vi "Dialog Box - Three Button.vi"(5 "Key Focus":enum16{"None", "1", "2", "3"}(ring), 6 "Button Text":T1={"Button 1"="Yes", "Button 2"="No", "Button 3"="Cancel"}, 7 "Timeout (Seconds)":i16=-1, 8 "error in (no error)":errorcluster, 11 "Text":string) -> (0 "error out":errorcluster, 1 "Button 3":bool, 2 "Button 2":bool, 3 "Button 1":bool, 4 "Timeout":bool)   [LabVIEW 2011]
doc: "Displays a simple two button dialog box.\n\nA timeout can be set. If no timeout is defined then the dialog will wait forever.\nThe text for each button can be set.\nEither button can receive key focus."
panel:
  in  "Button Three":bool
  in  "Button Two":bool
  in  "Button One":bool
  out "String":string
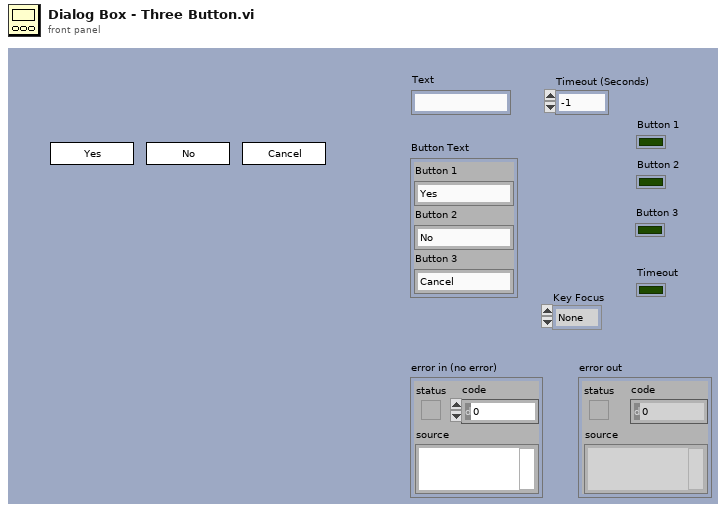
[diagram p1: front panel]
types:
  T1 = cluster{"Button 1":string, "Button 2":string, "Button 3":string}
  T2 = enum32{"Invalid", "Default", "Floating", "Floating/Auto-Hide", "Modal"}
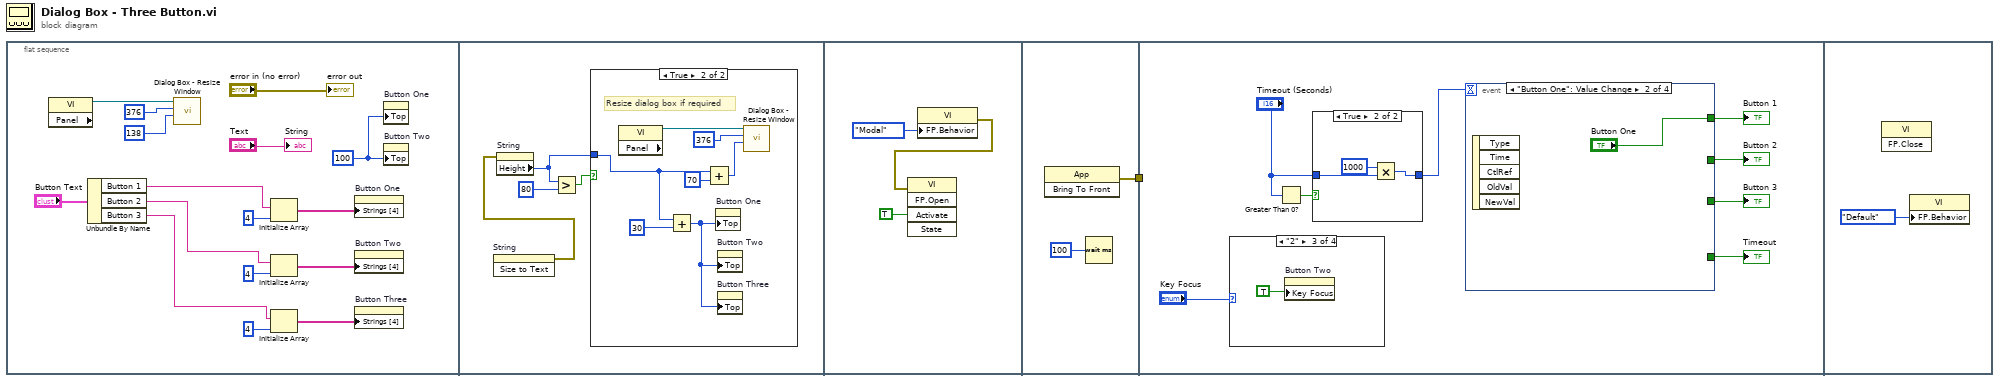
[diagram p0: block diagram]
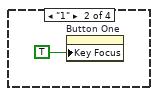
[diagram p4: hidden frame]
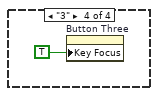
[diagram p5: hidden frame]
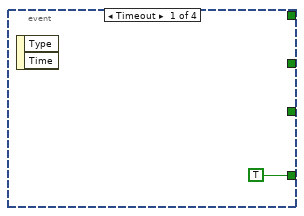
[diagram p6: hidden frame]
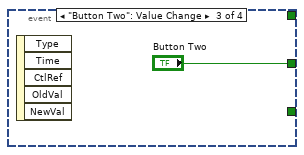
[diagram p7: hidden frame]
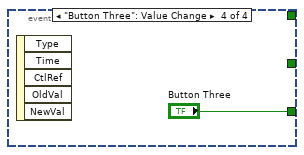
[diagram p8: hidden frame]
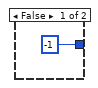
[diagram p9: hidden frame]
diagram:
  n1 = flat-sequence {
    tunnel: [w33] -> w1
    tunnel: w1 -> [_]
    frame #0 {
      w8 = 100 ("Position:Top")
      n2 = property class="VI" props=["Panel"]() -> (reference out=w11:refnum<vi>)  [unwired: 2 in, 2 out]
      n3 = Unbundle By Name("Button Text") -> ("Button 1"=w5:string, "Button 2"=w4:string, "Button 3"=w3:string)
      n4 = call "Dialog Box - Resize Window.vi"("Height"=i16 138, "Width"=i16 376, "reference"=w11) -> ()  [unwired: 8 in, 1 out]
      n5 = Initialize Array(w5, 4 ("dimension size")) -> (w12:string[])
      n6 = Initialize Array(w4, 4 ("dimension size")) -> (w13:string[])
      n7 = Initialize Array(w3, 4 ("dimension size")) -> (w2:string[])
      n8 = property on="Button One" class="Bool"("Strings [4]"=w12) -> ()  [unwired: 2 in, 2 out]
      n9 = property on="Button Two" class="Bool"("Strings [4]"=w13) -> ()  [unwired: 2 in, 2 out]
      n10 = property on="Button Three" class="Bool"("Strings [4]"=w2) -> ()  [unwired: 2 in, 2 out]
      n11 = property on="Button One" class="Bool"("Top"=w8) -> ()  [unwired: 2 in, 2 out]
      n12 = property on="Button Two" class="Bool"("Top"=w8) -> ()  [unwired: 2 in, 2 out]
      "String" <- "Text"
      "error out" <- "error in (no error)"
    }
    frame #1 {
      n13 = invoke on="String" class="Str" method="Size to Text"() -> (error out=w21:errorcluster)  [unwired: 3 in, 2 out]
      n14 = property on="String" class="Str"(error in=w21) -> ("Height"=w20:u32)  [unwired: 1 in, 2 out]
      n15 = Greater?(x=w20, y=u32 80) -> (0:w19:bool)
      n16 = case shown="True" w19 {
        tunnel: w20 -> [_ w24]
        frame False {
        }
        frame True {
          # "Resize dialog box if required"
          n17 = property class="VI" props=["Panel"]() -> (reference out=w28:refnum<vi>)  [unwired: 2 in, 2 out]
          n18 = Add(x=w24, y=u32 30) -> (x+y=w22:u32)
          n19 = Add(x=w24, y=u32 70) -> (x+y=w26:u32)
          n20 = property on="Button One" class="Bool"("Top"=w22) -> ()  [unwired: 2 in, 2 out]
          n21 = property on="Button Two" class="Bool"("Top"=w22) -> ()  [unwired: 2 in, 2 out]
          n22 = property on="Button Three" class="Bool"("Top"=w22) -> ()  [unwired: 2 in, 2 out]
          n23 = call "Dialog Box - Resize Window.vi"("Height"=w26, "Width"=i16 376, "reference"=w28) -> ()  [unwired: 8 in, 1 out]
        }
      }
    }
    frame #2 {
      n24 = property class="VI"("FP.Behavior"=T2."Modal" ("Front Panel Window:Behavior")) -> (error out=w29:errorcluster)  [unwired: 2 in, 1 out]
      n25 = invoke class="VI" method="FP.Open"(error in=w29, "Activate"=TRUE ("Activate?")) -> ()  [unwired: 3 in, 5 out]
    }
    frame #3 {
      n26 = invoke class="App" method="Bring To Front"() -> (error out=w33:errorcluster)  [unwired: 3 in, 2 out]
      n27 = Wait (ms)(milliseconds to wait=u32 100) -> ()  [unwired: 1 out]
    }
    frame #4 {
      n28 = case shown="\"2\"" "Key Focus" {
        frame "None" {
        }
        frame "1" {
          n29 = property on="Button One" class="Bool"("Key Focus"=TRUE) -> ()  [unwired: 2 in, 2 out]
        }
        frame "2" {
          n30 = property on="Button Two" class="Bool"("Key Focus"=TRUE) -> ()  [unwired: 2 in, 2 out]
        }
        frame "3" {
          n31 = property on="Button Three" class="Bool"("Key Focus"=TRUE) -> ()  [unwired: 2 in, 2 out]
        }
      }
      n32 = Greater Than 0?(x="Timeout (Seconds)") -> (x > 0?=w40:bool)
      n33 = case shown="True" w40 {
        tunnel: "Timeout (Seconds)" -> [_ w50]
        tunnel: [i16 -1 w51] -> w39
        frame False {
        }
        frame True {
          n34 = Multiply(x=i16 1000, y=w50) -> (x*y=w51:i16)
        }
      }
      n35 = event shown="[1] \"Button One\": Value Change" {
        selector: _ -> [_ _ _ _]
        dyn-events: _ -> [_ _ _ _]
        timeout: w39 -> [_ _ _ _]
        tunnel: [_ "Button One" _ _] -> w38
        tunnel: [_ _ "Button Two" _] -> w37
        tunnel: [TRUE _ _ _] -> w36
        tunnel: [_ _ _ "Button Three"] -> w34
        event Timeout {
          n36 = event-data() -> ()  [unwired: 1 in, 2 out]
        }
        event "Button One": Value Change {
          n37 = event-data() -> ()  [unwired: 1 in, 5 out]
        }
        event "Button Two": Value Change {
          n38 = event-data() -> ()  [unwired: 1 in, 5 out]
        }
        event "Button Three": Value Change {
          n39 = event-data() -> ()  [unwired: 1 in, 5 out]
        }
      }
      "Button 1" <- w38
      "Button 2" <- w37
      "Timeout" <- w36
      "Button 3" <- w34
    }
    frame #5 {
      n40 = invoke class="VI" method="FP.Close"() -> ()  [unwired: 3 in, 3 out]
      n41 = property class="VI"("FP.Behavior"=T2."Default" ("Front Panel Window:Behavior")) -> ()  [unwired: 2 in, 2 out]
    }
  }
